vi "3b.vi"() -> ()   [LabVIEW 2015]
panel:
  in  "Cluster":cluster{"Array":dbl[][]}
  out "Waveform Graph 3":dbl[](graph)
  out "Waveform Graph 2":dbl[](graph)
  out "Waveform Graph":dbl[](graph)
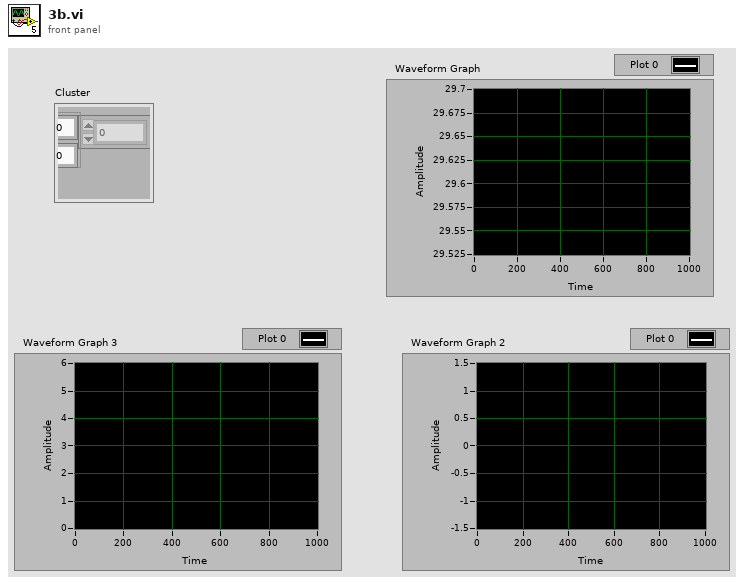
[diagram p1: front panel]
types:
  T1 = enum16{"open", "replace", "create", "open or create", "replace or create", "replace or create with confirmation"}
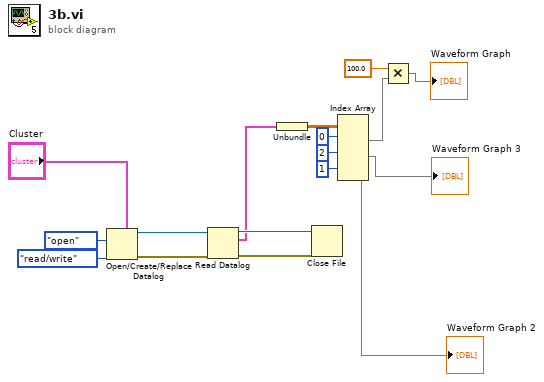
[diagram p0: block diagram]
diagram:
  n1 = Open/Create/Replace Datalog(5:"Cluster", 9:enum16{"read/write", "read-only", "write-only"}."read/write" ("access (0:read/write)"), 10:T1."open" ("operation (0:open)")) -> (0:w14:errorcluster, 3:w12:refnum<k1>)  [unwired: 3 in, 1 out]
  n2 = Read Datalog(4:w14, 7:w12) -> (0:w13:errorcluster, 2:w10:cluster{"Array":dbl[][]}, 3:w11:refnum<k1>)  [unwired: 1 in]
  n3 = Unbundle(w10) -> ("Array"=w9:dbl[][])
  n4 = Close File(refnum=w11, error in=w13) -> ()  [unwired: 2 out]
  n5 = Index Array(array=w9, index (row) #1=0 ("index (row)"), index (row) #2=2 ("index (row)"), index (row) #3=1 ("index (row)")) -> (element #1=w5:dbl[], element #2=→"Waveform Graph 3":dbl[], element #3=→"Waveform Graph 2":dbl[])  [unwired: 3 in]
  n6 = Multiply(x=100.0, y=w5) -> (x*y=→"Waveform Graph":dbl[])
